vi "Build NT RPC Response.vi"(8 "error in (no error)":errorcluster, 11 "RPC Info":T1) -> (0 "error out":errorcluster, 3 "VI out":refnum<vi>)   [LabVIEW 2017]
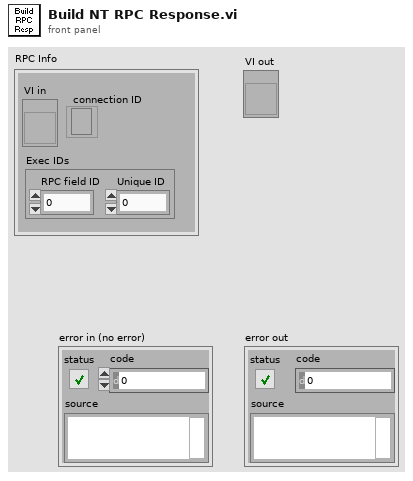
[diagram p1: front panel]
types:
  T1 = cluster{"VI in":refnum<vi>, "connection ID":refnum<k5>, "Exec IDs":cluster{"RPC field ID":u16, "Unique ID":u16}}
  T2 = typedef "Field Data.ctl" = cluster{"Dbl":dbl, "String":string, "Type":T3, "Boolean":bool, "Sequence #":T4, "Flags":u8}
  T3 = typedef "Field Type.ctl" = enum8{"Invalid", "Bool", "Numeric", "String", "Raw", "Boolean Array", "Numeric Array", "String Array", "RPC"}
  T4 = typedef "Sequence.ctl" = u16
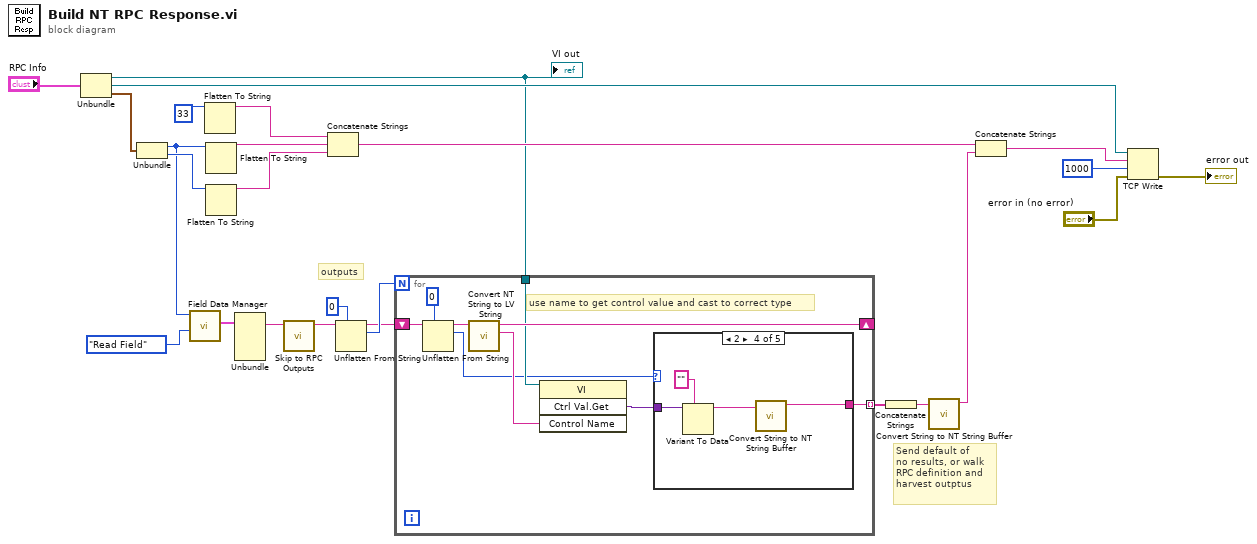
[diagram p0: block diagram]
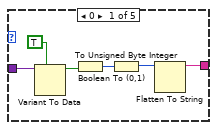
[diagram p2: hidden frame]
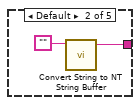
[diagram p3: hidden frame]
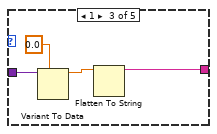
[diagram p4: hidden frame]
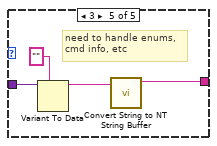
[diagram p5: hidden frame]
diagram:
  # "outputs"
  # "Send default of\nno results, or walk\nRPC definition and\nharvest outptus"
  n1 = Unbundle("RPC Info") -> ("VI in"=w1:refnum<vi>, "connection ID"=w17:refnum<k5>, "Exec IDs"=w19:cluster{"RPC field ID":u16, "Unique ID":u16})
  "VI out" <- w1
  n2 = Unbundle(w19) -> ("RPC field ID"=w13:u16, "Unique ID"=w23:u16)
  n3 = call <vilib>:"Field Data Manager.vi"("Operation"=enum16{"Update Field", "Read Field"}."Read Field", "Field ID"=w13) -> ("Field Value Out"=w12:T2)  [unwired: 8 in, 1 out]
  n4 = Flatten To String(anything=u8 33 ("bytes to read")) -> (data string=w24:string)  [unwired: 3 in, 2 out]
  n5 = Flatten To String(anything=w13) -> (data string=w22:string)  [unwired: 3 in, 2 out]
  n6 = Flatten To String(anything=w23) -> (data string=w21:string)  [unwired: 3 in, 2 out]
  n7 = Unbundle(w12) -> ("String"=w8:string)  [unwired: 5 out]
  n8 = call <vilib>:"Skip to RPC Outputs.vi"("String in"=w8) -> ("String out"=w7:string)  [unwired: 8 in, 2 out]
  n9 = Concatenate Strings(w24, w22, w21) -> (w4:string)
  n10 = Unflatten From String(type=u8 0 ("bytes to read"), binary string=w7) -> (rest of the binary string=w9:string, value=w10:u8)  [unwired: 3 in, 1 out]
  n11 = for {
    N: w10 -> [_]
    shift-right: [w31] -> _
    shift-left: w9 -> [w32]
    tunnel: w1 -> [w30]
    tunnel: [w27] -> w6 mode=indexing
    # "use name to get control value and cast to correct type"
    n12 = Unflatten From String(type=u8 0 ("bytes to read"), binary string=w32) -> (rest of the binary string=w34:string, value=w26:u8)  [unwired: 3 in, 1 out]
    n13 = call <vilib>:"Convert NT String to LV String.vi"("Buffer in"=w34) -> ("String Contents"=w29:string, "Remaining String"=w31:string)  [unwired: 8 in, 1 out]
    n14 = invoke class="VI" method="Ctrl Val.Get"(reference=w30, "Control Name"=w29) -> ("Get Control Value Variant"=w28:variant)  [unwired: 2 in, 3 out]
    n15 = case shown="2" w26 {
      tunnel: w28 -> [w40 _ w46 w50 w54]
      tunnel: [w35 w41 w43 w47 w51] -> w27
      frame 0 {
        n16 = Variant To Data(type=TRUE, Variant=w40) -> (data=w36:bool)  [unwired: 1 in, 1 out]
        n17 = Boolean To (0,1)(Boolean=w36) -> (0, 1=w37:i16)
        n18 = To Unsigned Byte Integer(number=w37) -> (unsigned 8bit integer=w38:u8)
        n19 = Flatten To String(anything=w38) -> (data string=w35:string)  [unwired: 3 in, 2 out]
      }
      frame Default {
        n20 = call <vilib>:"Convert String to NT String Buffer.vi"("LV Buffer"="") -> ("NT Buffer"=w41:string)  [unwired: 10 in]
      }
      frame 1 {
        n21 = Variant To Data(type=0.0, Variant=w46) -> (data=w44:dbl)  [unwired: 1 in, 1 out]
        n22 = Flatten To String(anything=w44) -> (data string=w43:string)  [unwired: 3 in, 2 out]
      }
      frame 2 {
        n23 = Variant To Data(type="", Variant=w50) -> (data=w48:string)  [unwired: 1 in, 1 out]
        n24 = call <vilib>:"Convert String to NT String Buffer.vi"("LV Buffer"=w48) -> ("NT Buffer"=w47:string)  [unwired: 10 in]
      }
      frame 3 {
        # "need to handle enums,\ncmd info, etc"
        n25 = Variant To Data(type="", Variant=w54) -> (data=w52:string)  [unwired: 1 in, 1 out]
        n26 = call <vilib>:"Convert String to NT String Buffer.vi"("LV Buffer"=w52) -> ("NT Buffer"=w51:string)  [unwired: 10 in]
      }
    }
  }
  n27 = Concatenate Strings(w6) -> (w5:string)
  n28 = call <vilib>:"Convert String to NT String Buffer.vi"("LV Buffer"=w5) -> ("NT Buffer"=w2:string)  [unwired: 10 in]
  n29 = Concatenate Strings(w4, w2) -> (w3:string)
  n30 = TCP Write(connection ID=w17, data in=w3, error in (no error)="error in (no error)", 9:1000 ("timeout ms (25000)")) -> (error out=→"error out":errorcluster)  [unwired: 2 out]
